vi "Save_PLC (SubVI).vi"(8 "error in (no error)":errorcluster, 10 "PLC":map{string, dbl}(c390), 11 "Refnum in":refnum<k34>) -> (0 "error out":errorcluster, 3 "Refnum out":refnum<k34>)   [LabVIEW 2024]
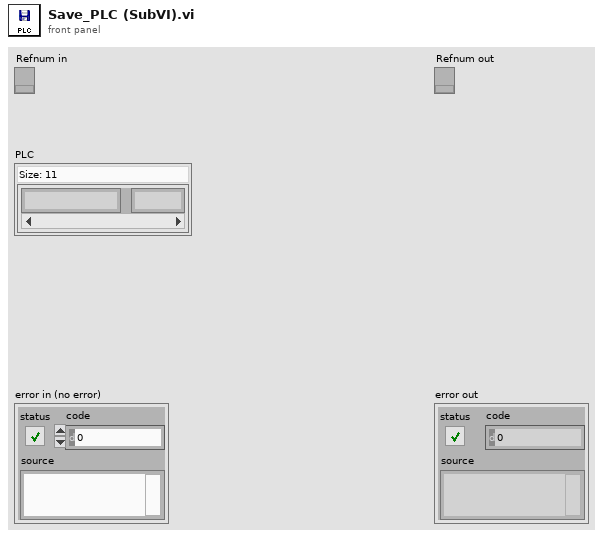
[diagram p1: front panel]
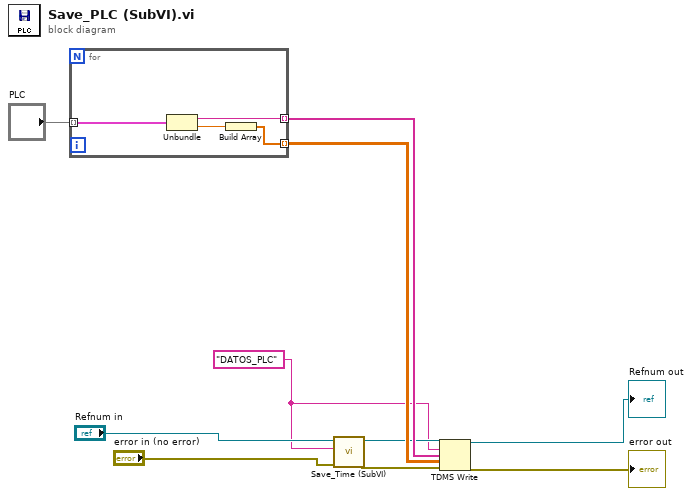
[diagram p0: block diagram]
diagram:
  w1 = "DATOS_PLC" ("group name in (Untitled)")
  n1 = for {
    tunnel: "PLC" -> [w14] mode=indexing
    tunnel: [w13] -> w7 mode=indexing
    tunnel: [w11] -> w8 mode=indexing
    n2 = Unbundle(w14) -> (w13:string, w12:dbl)
    n3 = Build Array(w12) -> (w11:dbl[])
  }
  n4 = call "Save_Time (SubVI).vi"("error in (no error)"="error in (no error)", "group name in (Untitled)"=w1, "Refnum in"="Refnum in") -> ("error out"=w2:errorcluster, "Refnum out"=w3:refnum<k34>)  [unwired: 7 in]
  n5 = TDMS Write(0:w3, 5:w1, 7:w7, 9:w8, 11:w2) -> (4:→"Refnum out":refnum<k34>, 15:→"error out":errorcluster)  [unwired: 1 in, 2 out]
